vi "AssembleSiPCB.vi"() -> ()   [LabVIEW 2019]
uses:
  Control 1.ctl
panel:
  in  "SyringeX":dbl=384.897 format="%#_13g"
  in  "SyringeY":dbl=891.926 format="%#_13g"
  in  "SyringeZ":dbl=77.153
  in  "VISA resource name":refnum<visa-resource-name>="COM5"
  in  "GlPatternSi":path=path "C:/Users/TTUHEP/Documents/LabVIEW/Data/Patterns/PCB_base_Dec21_rotated2_Combined.ngc"
  in  "GlPatternPCB":path=path "C:/Users/TTUHEP/Documents/LabVIEW/Data/Patterns/Nonstepped_09-22-2021_rotated2_Version10_2_Combined.ngc"
  in  "GoHome":bool
  in  "PCBPositions":path=path "C:/Users/TTUHEP/Documents/LabVIEW/Data/AssemblyIO_logs/PCBPositions.txt"
  in  "PUT_Positions":path=path "C:/Users/TTUHEP/Documents/LabVIEW/Data/AssemblyIO_logs/PUT2_Positions.txt"
  in  "SiPositions":path=path "C:/Users/TTUHEP/Documents/LabVIEW/Data/AssemblyIO_logs/SensorPositions.txt"
  in  "BasePlatePositions":path=path "C:/Users/TTUHEP/Documents/LabVIEW/Data/AssemblyIO_logs/BaseplatePositions.txt"
  in  "PressureSiPCB":T1[](array[typedef])=[15.0, 14.0, 8.0, 0.0]
  in  "PressureBPSi":dbl[](array[numeric])=[30.0, 15.0, 0.0, 0.0]
  in  "Glue":bool
  in  "SiAssemblyVacs":u64[](array[numeric])=[2162752, 2162752, 35717184, 52428864, 2098240]
  in  "PCBAssemblyVacs":u64[](array[numeric])=[2162752, 2162752, 35717184, 52428864, 2098240]
  in  "GoToBP":bool
  in  "PickSiPCB":bool
  in  "AssmbType":enum16{"Sensor", "PCB"}(ring)
  in  "GoToSenPCB":bool
  in  "DropTool":bool
  in  "PickTool":bool
  in  "GoToToolPos":bool
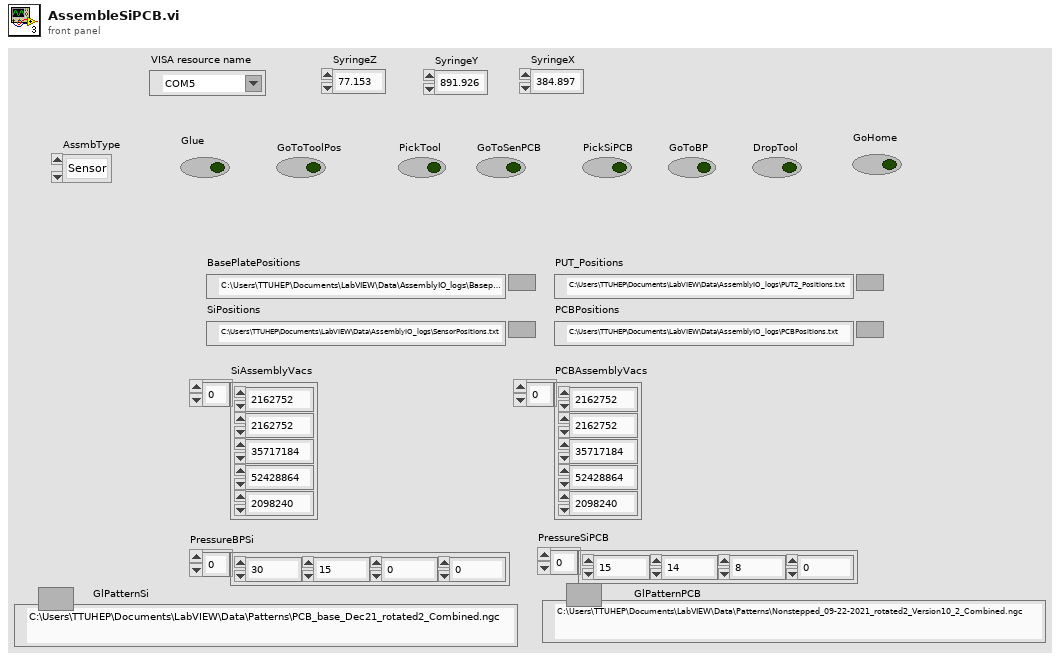
[diagram p1: front panel]
types:
  T1 = typedef "Control 1.ctl" = dbl
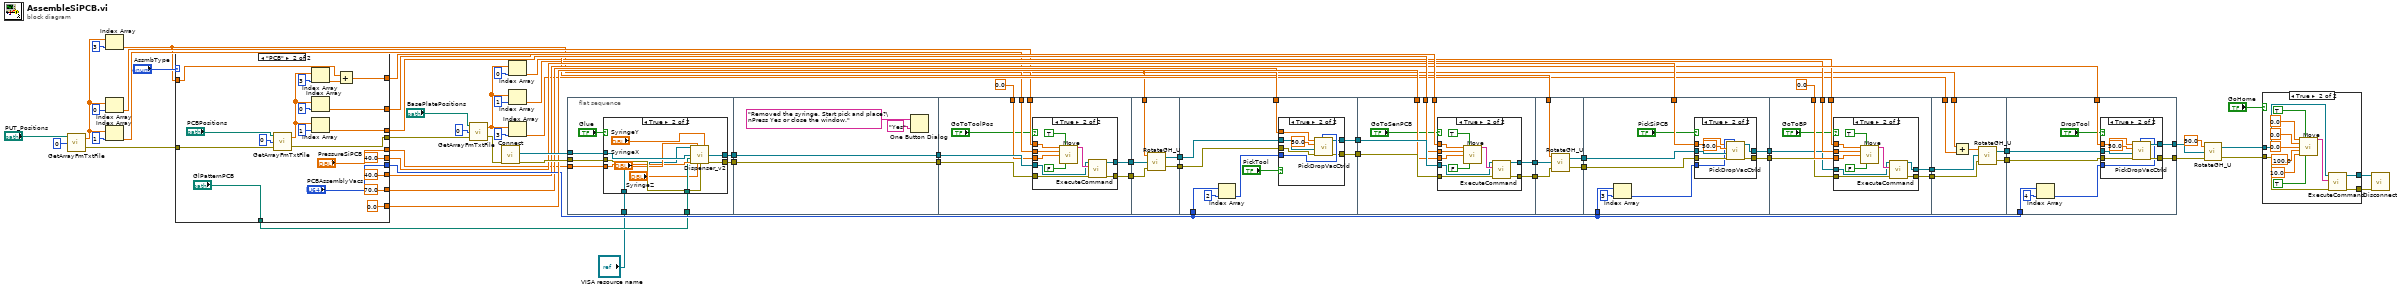
[diagram p0: block diagram]
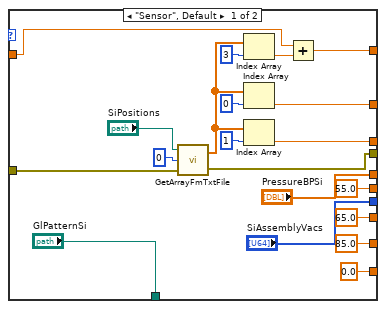
[diagram p3: hidden frame]
diagram:
  n1 = call "GetArrayFmTxtFile.vi"("LineNo."=0, "TextFile"="PUT_Positions") -> ("error out"=w13:errorcluster, "Array"=w21:dbl[])  [unwired: 1 in]
  n2 = Index Array(array=w21, index=3) -> (element=w14:dbl)
  n3 = Index Array(array=w21, index=0) -> (element=w17:dbl)
  n4 = Index Array(array=w21, index=1) -> (element=w16:dbl)
  n5 = case shown="\"PCB\"" "AssmbType" {
    tunnel: [w76 w93] -> w60
    tunnel: [w75 w92] -> w59
    tunnel: [0.0 0.0] -> w58
    tunnel: ["SiAssemblyVacs" "PCBAssemblyVacs"] -> w55
    tunnel: [85.0 ("Z") 70.0 ("Z")] -> w54
    tunnel: [55.0 ("Z") 40.0 ("Z")] -> w53
    tunnel: [65.0 ("Z") 40.0 ("Z")] -> w52
    tunnel: w14 -> [w81 w101]
    tunnel: [w80 w100] -> w45
    tunnel: ["PressureBPSi" "PressureSiPCB"] -> w31
    tunnel: w13 -> [w71 w96]
    tunnel: [w70 w95] -> w12
    tunnel: ["GlPatternSi" "GlPatternPCB"] -> w2
    frame "Sensor", Default {
      n6 = call "GetArrayFmTxtFile.vi"("error in"=w71, "LineNo."=0, "TextFile"="SiPositions") -> ("error out"=w70:errorcluster, "Array"=w72:dbl[])
      n7 = Index Array(array=w72, index=3) -> (element=w73:dbl)
      n8 = Index Array(array=w72, index=0) -> (element=w76:dbl)
      n9 = Index Array(array=w72, index=1) -> (element=w75:dbl)
      n10 = Add(x=w81, y=w73) -> (x+y=w80:dbl)
    }
    frame "PCB" {
      n11 = call "GetArrayFmTxtFile.vi"("error in"=w96, "LineNo."=0, "TextFile"="PCBPositions") -> ("error out"=w95:errorcluster, "Array"=w94:dbl[])
      n12 = Index Array(array=w94, index=3) -> (element=w90:dbl)
      n13 = Index Array(array=w94, index=0) -> (element=w93:dbl)
      n14 = Index Array(array=w94, index=1) -> (element=w92:dbl)
      n15 = Add(x=w101, y=w90) -> (x+y=w100:dbl)
    }
  }
  n16 = call "GetArrayFmTxtFile.vi"("error in"=w12, "LineNo."=0, "TextFile"="BasePlatePositions") -> ("error out"=w11:errorcluster, "Array"=w26:dbl[])
  n17 = call "Connect.vi"("error in (no error)"=w11) -> ("error out"=w64:errorcluster, "controller"=w65:refnum<k24>)  [unwired: 9 in]
  n18 = Index Array(array=w26, index=0) -> (element=w30:dbl)
  n19 = Index Array(array=w26, index=1) -> (element=w29:dbl)
  n20 = Index Array(array=w26, index=3) -> (element=w27:dbl)
  n21 = flat-sequence {
    tunnel: [w111] -> w35
    tunnel: [w112] -> w33
    tunnel: w31 -> [w108]
    tunnel: w65 -> [w110]
    tunnel: w64 -> [w113]
    tunnel: w2 -> [w107]
    tunnel: "VISA resource name" -> [w106]
    tunnel: w35 -> [w129]
    tunnel: [w129] -> w34
    tunnel: w33 -> [w128]
    tunnel: [w128] -> w32
    tunnel: w17 -> [w135]
    tunnel: w16 -> [w134]
    tunnel: 0.0 -> [w133]
    tunnel: w34 -> [w137]
    tunnel: w32 -> [w136]
    tunnel: [w132] -> w51
    tunnel: [w131] -> w50
    tunnel: w51 -> [w154]
    tunnel: [w153] -> w37
    tunnel: w50 -> [w152]
    tunnel: [w151] -> w36
    tunnel: w14 -> [w150]
    tunnel: w37 -> [w163]
    tunnel: w36 -> [w162]
    tunnel: [w161] -> w63
    tunnel: [w160] -> w62
    tunnel: w55 -> [w157]
    tunnel: w54 -> [w156]
    tunnel: w63 -> [w177]
    tunnel: [w178] -> w49
    tunnel: w62 -> [w179]
    tunnel: [w180] -> w47
    tunnel: w60 -> [w176]
    tunnel: w59 -> [w175]
    tunnel: w58 -> [w174]
    tunnel: w49 -> [w197]
    tunnel: [w194] -> w48
    tunnel: w47 -> [w196]
    tunnel: [w195] -> w46
    tunnel: w45 -> [w193]
    tunnel: w48 -> [w205]
    tunnel: w46 -> [w206]
    tunnel: [w204] -> w57
    tunnel: [w203] -> w56
    tunnel: w55 -> [w200]
    tunnel: w53 -> [w199]
    tunnel: w57 -> [w220]
    tunnel: [w217] -> w44
    tunnel: w56 -> [w219]
    tunnel: [w218] -> w42
    tunnel: w30 -> [w223]
    tunnel: w29 -> [w222]
    tunnel: 0.0 -> [w221]
    tunnel: w44 -> [w241]
    tunnel: [w240] -> w43
    tunnel: w42 -> [w242]
    tunnel: [w239] -> w41
    tunnel: w14 -> [w237]
    tunnel: w27 -> [w236]
    tunnel: [w248] -> w40
    tunnel: w43 -> [w250]
    tunnel: [w249] -> w39
    tunnel: w55 -> [w246]
    tunnel: w52 -> [w244]
    tunnel: w41 -> [w251]
    frame #0 {
      n22 = case shown="True" "Glue" {
        tunnel: w113 -> [w114 w125]
        tunnel: [w114 w124] -> w112
        tunnel: [w115 w123] -> w111
        tunnel: w110 -> [w115 w122]
        tunnel: w108 -> [_ w119]
        tunnel: w107 -> [_ w118]
        tunnel: w106 -> [_ w117]
        frame False {
        }
        frame True {
          n23 = call "Dispenser_v2.vi"("VISA resource name"=w117, "X"="SyringeX", "Y"="SyringeY", "controller in"=w122, "Path"=w118, "Pressure"=w119, "Z"="SyringeZ", "error in (no error)"=w125) -> ("controller out"=w123:refnum<k24>, "error out"=w124:errorcluster)  [unwired: 3 in, 3 out]
        }
      }
    }
    frame #1 {
      n24 = One Button Dialog(message="Removed the syringe. Start pick and place?\nPress Yes or close the window.", button name ("OK")="Yes") -> ()  [unwired: 1 out]
    }
    frame #2 {
      n25 = case shown="True" "GoToToolPos" {
        tunnel: w137 -> [w139 w146]
        tunnel: w136 -> [w138 w145]
        tunnel: [w138 w144] -> w131
        tunnel: [w139 w143] -> w132
        tunnel: w135 -> [_ w142]
        tunnel: w134 -> [_ w141]
        tunnel: w133 -> [_ w140]
        frame False {
        }
        frame True {
          n26 = call "Move.vi"("X"=w142, "Absolute"=TRUE, "Y"=w141, "Z"=w140, "Move Z first"=FALSE) -> ("Position Gcode"=w147:string)  [unwired: 10 in]
          n27 = call "ExecuteCommand.vi"("error in (no error)"=w145, "Command Code"=w147, "controller in"=w146) -> ("error out"=w144:errorcluster, "controller out"=w143:refnum<k24>)  [unwired: 6 in, 1 out]
        }
      }
    }
    frame #3 {
      n28 = call "RotateGH_U.vi"("error in (no error)"=w152, "controller in"=w154, "U"=w150) -> ("error out"=w151:errorcluster, "controller out"=w153:refnum<k24>)
    }
    frame #4 {
      n29 = Index Array(array=w157, index=2) -> (element=w158:u64)
      n30 = case shown="True" "PickTool" {
        tunnel: w163 -> [w165 w171]
        tunnel: w162 -> [w164 w170]
        tunnel: w158 -> [_ w169]
        tunnel: [w165 w168] -> w161
        tunnel: [w164 w167] -> w160
        tunnel: w156 -> [_ w166]
        frame False {
        }
        frame True {
          n31 = call "PickDropVacCtrld.vi"("VacuumState"=w169, "error in (no error)"=w170, "controller in"=w171, "Zspeed"=50.0, "Z"=w166) -> ("error out"=w167:errorcluster, "controller out"=w168:refnum<k24>)  [unwired: 5 in]
        }
      }
    }
    frame #5 {
      n32 = case shown="True" "GoToSenPCB" {
        tunnel: [w182 w183] -> w180
        tunnel: w179 -> [w182 w185]
        tunnel: [w181 w184] -> w178
        tunnel: w177 -> [w181 w186]
        tunnel: w176 -> [_ w189]
        tunnel: w175 -> [_ w188]
        tunnel: w174 -> [_ w187]
        frame False {
        }
        frame True {
          n33 = call "Move.vi"("X"=w189, "Absolute"=TRUE, "Y"=w188, "Z"=w187, "Move Z first"=FALSE) -> ("Position Gcode"=w190:string)  [unwired: 10 in]
          n34 = call "ExecuteCommand.vi"("error in (no error)"=w185, "Command Code"=w190, "controller in"=w186) -> ("error out"=w183:errorcluster, "controller out"=w184:refnum<k24>)  [unwired: 6 in, 1 out]
        }
      }
    }
    frame #6 {
      n35 = call "RotateGH_U.vi"("error in (no error)"=w196, "controller in"=w197, "U"=w193) -> ("error out"=w195:errorcluster, "controller out"=w194:refnum<k24>)
    }
    frame #7 {
      n36 = Index Array(array=w200, index=3) -> (element=w201:u64)
      n37 = case shown="True" "PickSiPCB" {
        tunnel: w205 -> [w208 w214]
        tunnel: w206 -> [w207 w213]
        tunnel: [w208 w212] -> w203
        tunnel: [w207 w211] -> w204
        tunnel: w201 -> [_ w210]
        tunnel: w199 -> [_ w209]
        frame False {
        }
        frame True {
          n38 = call "PickDropVacCtrld.vi"("VacuumState"=w210, "error in (no error)"=w213, "controller in"=w214, "Zspeed"=50.0, "Z"=w209) -> ("error out"=w211:errorcluster, "controller out"=w212:refnum<k24>)  [unwired: 5 in]
        }
      }
    }
    frame #8 {
      n39 = case shown="True" "GoToBP" {
        tunnel: [w225 w229] -> w217
        tunnel: w220 -> [w225 w231]
        tunnel: [w224 w230] -> w218
        tunnel: w219 -> [w224 w232]
        tunnel: w223 -> [_ w228]
        tunnel: w222 -> [_ w227]
        tunnel: w221 -> [_ w226]
        frame False {
        }
        frame True {
          n40 = call "Move.vi"("X"=w228, "Absolute"=TRUE, "Y"=w227, "Z"=w226, "Move Z first"=FALSE) -> ("Position Gcode"=w233:string)  [unwired: 10 in]
          n41 = call "ExecuteCommand.vi"("error in (no error)"=w231, "Command Code"=w233, "controller in"=w232) -> ("error out"=w229:errorcluster, "controller out"=w230:refnum<k24>)  [unwired: 6 in, 1 out]
        }
      }
    }
    frame #9 {
      n42 = Add(x=w237, y=w236) -> (x+y=w238:dbl)
      n43 = call "RotateGH_U.vi"("error in (no error)"=w241, "controller in"=w242, "U"=w238) -> ("error out"=w240:errorcluster, "controller out"=w239:refnum<k24>)
    }
    frame #10 {
      n44 = Index Array(array=w246, index=4) -> (element=w245:u64)
      n45 = case shown="True" "DropTool" {
        tunnel: w251 -> [w253 w259]
        tunnel: w250 -> [w252 w258]
        tunnel: [w253 w257] -> w248
        tunnel: [w252 w256] -> w249
        tunnel: w245 -> [_ w255]
        tunnel: w244 -> [_ w254]
        frame False {
        }
        frame True {
          n46 = call "PickDropVacCtrld.vi"("VacuumState"=w255, "error in (no error)"=w258, "controller in"=w259, "Zspeed"=50.0, "Z"=w254) -> ("error out"=w256:errorcluster, "controller out"=w257:refnum<k24>)  [unwired: 5 in]
        }
      }
    }
  }
  n47 = call "RotateGH_U.vi"("error in (no error)"=w39, "controller in"=w40, "U"=90.0) -> ("error out"=w10:errorcluster, "controller out"=w9:refnum<k24>)
  n48 = case shown="True" "GoHome" {
    tunnel: w10 -> [w261 w266]
    tunnel: w9 -> [w262 w265]
    tunnel: [w262 w264] -> w8
    tunnel: [w261 w263] -> w7
    frame False {
    }
    frame True {
      n49 = call "Move.vi"("X"=0.0, "Absolute"=TRUE, "Y"=0.0, "Z"=0.0, "SpeedXY (mm/s)"=100.0, "SpeedZ (mm/s)"=10.0, "Move Z first"=TRUE) -> ("Position Gcode"=w267:string)  [unwired: 8 in]
      n50 = call "ExecuteCommand.vi"("error in (no error)"=w266, "Command Code"=w267, "controller in"=w265) -> ("error out"=w263:errorcluster, "controller out"=w264:refnum<k24>)  [unwired: 6 in, 1 out]
    }
  }
  n51 = call "Disconnect.vi"("error in (no error)"=w7, "controller"=w8) -> ()  [unwired: 9 in, 1 out]
